vi "MLS Sequence Waveform.vi"(6 "sampling info":cluster{"Fs":dbl, "#s":dbl}={"Fs"=1000.0, "#s"=1000.0} {"Fs" format="%.2p"}, 7 "reset signal":bool, 8 "error in (no error)":errorcluster, 10 "seed":i32=-1, 11 "polynomial order":i32=31) -> (0 "error out":errorcluster, 3 "signal out":waveform(u8))   [LabVIEW 2020, in "NI_MABase.lvlib"]
doc: "Generates a maximum length sequence of ones and zeros using a modulo-2 primitive polynomial of order <B>polynomial order</B>."
uses:
  NI_MABase.lvlib
  NI_AALBase.lvlib
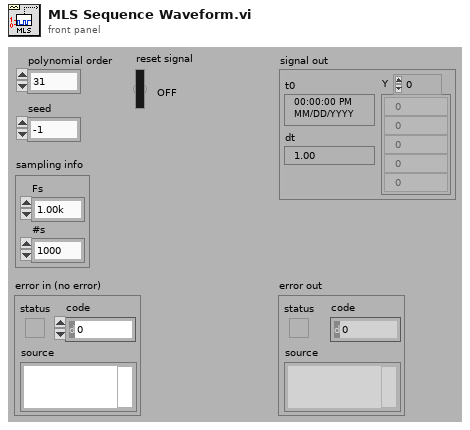
[diagram p1: front panel]
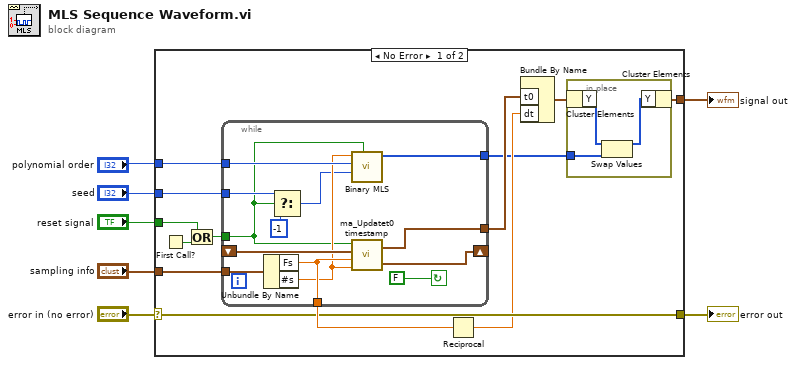
[diagram p0: block diagram]
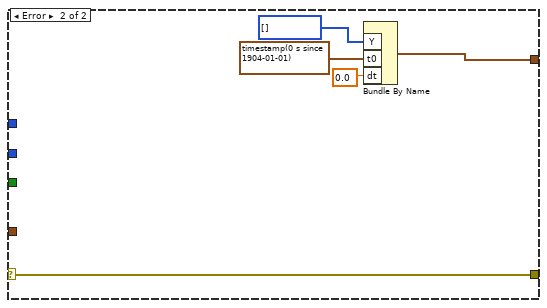
[diagram p2: hidden frame]
diagram:
  n1 = case shown="No Error" "error in (no error)" {
    selector: "error in (no error)" -> [w16 w41]
    tunnel: [w16 w41] -> w7
    tunnel: "sampling info" -> [w20 _]
    tunnel: "polynomial order" -> [w18 _]
    tunnel: "seed" -> [w17 _]
    tunnel: [w8 w40] -> w2
    tunnel: "reset signal" -> [w11 _]
    frame No Error {
      n2 = First Call?() -> (First Call?: T/F=w13:bool)
      n3 = Or(x=w11, y=w13) -> (x .or. y?=w12:bool)
      n4 = while {
        tunnel: w12 -> [w24]
        tunnel: w17 -> [w27]
        tunnel: w18 -> [w30]
        tunnel: [w31] -> w19
        tunnel: w20 -> [w32]
        tunnel: [w29] -> w9
        tunnel: [w34] -> w14
        shift-left: _ -> [w36]
        shift-right: [w35] -> _
        stop <- FALSE continue-if-true
        n5 = Unbundle By Name(w32) -> ("Fs"=w31:dbl, "#s"=w28:dbl)
        n6 = Select(t=w27, s=w24, f=-1) -> (s? t:f=w26:i32)
        n7 = call "Binary MLS.vi"("initialize?"=w24, "seed"=w26, "polynomial order"=w30, "samples"=w28) -> ("mls sequence"=w29:u8[])  [unwired: 6 in, 1 out]
        n8 = call "ma_Updatet0 timestamp.vi"("samples"=w28, "sampling rate (S/s)"=w31, "tf previous"=w36, "Reset Generation"=w24) -> ("tf new"=w35:timestamp, "t0"=w34:timestamp)
      }
      n9 = Reciprocal(x=w19) -> (1/x=w15:dbl)
      n10 = Bundle By Name("t0"=w14, "dt"=w15) -> (w10:waveform(u8))  [unwired: 1 out]
      n11 = in-place {
        in-place-border: w9 -> [w21]
        n12 = in-place-cluster #1(w10) -> ("Y"=w23:u8[])
        n13 = Swap Values(12:w23, 14:w21) -> (1:w22:u8[])  [unwired: 1 in, 1 out]
        n14 = in-place-cluster #1("Y"=w22) -> (w8:waveform(u8))
      }
    }
    frame Error {
      n15 = Bundle By Name("Y"=u8[] [], "t0"=timestamp(0 s since 1904-01-01), "dt"=0.0 ("t0")) -> (w40:waveform(u8))  [unwired: 1 out]
    }
  }
  "error out" <- w7
  "signal out" <- w2
